vi "send_frames.vi"(8 "error in":errorcluster, 10 "frame data":T1, 11 "TCP Network Connection in":refnum<k5>) -> (0 "error out":errorcluster)   [LabVIEW 2019, in "WebSocket Server Toolkit.lvlib"]
uses:
  WebSocket Server Toolkit.lvlib
  types/frame_data.ctl
  types/opcode.ctl
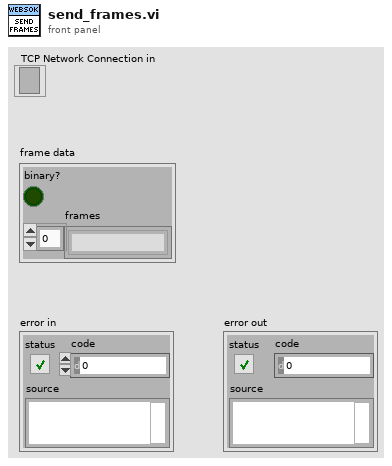
[diagram p1: front panel]
types:
  T1 = typedef "WebSocket Server Toolkit.lvlib/frame_data.ctl" = cluster{"binary?":bool, "frames":string[]}
  T2 = typedef "WebSocket Server Toolkit.lvlib/opcode.ctl" = u8
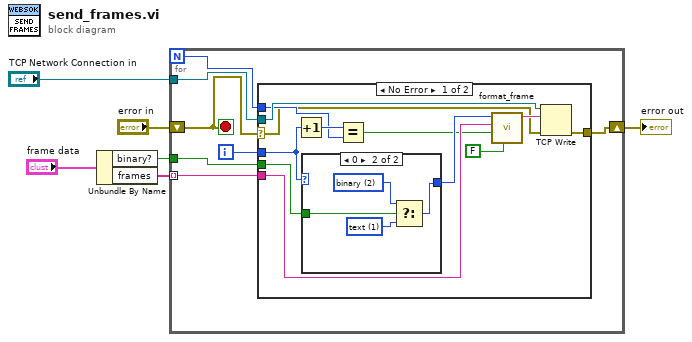
[diagram p0: block diagram]
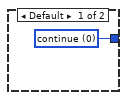
[diagram p2: hidden frame]
diagram:
  n1 = Unbundle By Name("frame data") -> ("binary?"=w4:bool, "frames"=w3:string[])
  n2 = for {
    N -> [w9]
    tunnel: "TCP Network Connection in" -> [w13]
    tunnel: w4 -> [w12]
    tunnel: w3 -> [w11] mode=indexing
    shift-right: [w8] -> w2
    shift-left: "error in" -> [w7]
    i -> [w10]
    stop <- w7 stop-if-true
    n3 = case shown="No Error" w7 {
      selector: w7 -> [w14 w31]
      tunnel: w13 -> [w25 _]
      tunnel: w12 -> [w22 _]
      tunnel: w11 -> [w21 _]
      tunnel: w10 -> [w20 _]
      tunnel: w9 -> [w18 _]
      tunnel: [w15 w31] -> w8
      frame No Error {
        n4 = Increment(x=w20) -> (x+1=w19:i32)
        n5 = case shown="0" w20 {
          tunnel: [w26 w28] -> w23
          tunnel: w22 -> [_ w27]
          frame Default {
            w26 = T2 0 items=["continue"=0, "text"=1, "binary"=2, "hangup"=8, "ping"=9, "pong"=10] ("opcode")
          }
          frame 0 {
            w29 = T2 1 items=["continue"=0, "text"=1, "binary"=2, "hangup"=8, "ping"=9, "pong"=10] ("opcode")
            w30 = T2 2 items=["continue"=0, "text"=1, "binary"=2, "hangup"=8, "ping"=9, "pong"=10] ("opcode")
            n6 = Select(t=w30, s=w27, f=w29) -> (s? t:f=w28:T2)
          }
        }
        n7 = Equal?(x=w19, y=w18) -> (x = y?=w17:bool)
        n8 = call "format_frame.vi"("mask?"=FALSE, "fin?"=w17, "data in"=w21, "opcode"=w23) -> ("frame data out"=w24:string)  [unwired: 7 in]
        n9 = TCP Write(connection ID=w25, data in=w24, error in (no error)=w14) -> (error out=w15:errorcluster)  [unwired: 1 in, 2 out]
      }
      frame Error {
      }
    }
  }
  "error out" <- w2
